vi "Target to Pixel.vi"(8 "Symbol":u32[][](array[colorbox]), 11 "Target Coordinates":dbl[](array[numeric])) -> (3 "Target Pixel":cluster{"X":i32, "Y":i32})   [LabVIEW 2018]
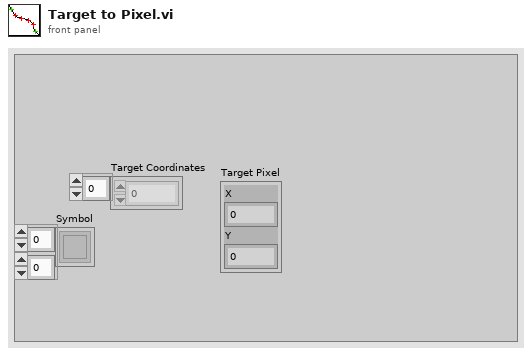
[diagram p1: front panel]
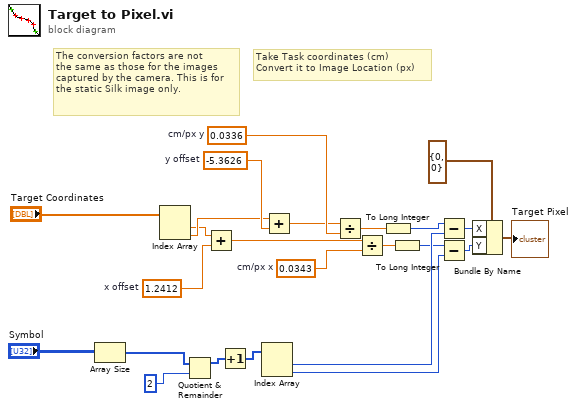
[diagram p0: block diagram]
diagram:
  w21 = 0.0336  # cm/px y
  w22 = 1.2412  # x offset
  w23 = 0.0343  # cm/px x
  w20 = -5.3626  # y offset
  # "The conversion factors are not \nthe same as those for the images\ncaptured by the camera. This is for\nthe static Silk image only."
  # "Take Task coordinates (cm)\nConvert it to Image Location (px)"
  n1 = Array Size(array="Symbol") -> (size(s)=w6:i32[])
  n2 = Index Array(array="Target Coordinates") -> (element #1=w1:dbl, element #2=w2:dbl)  [unwired: 2 in]
  n3 = Quotient & Remainder(x=w6, y=2) -> (x-y*floor(x/y)=w4:i32[])  [unwired: 1 out]
  n4 = Add(x=w1, y=w22) -> (x+y=w16:dbl)
  n5 = Increment(x=w4) -> (x+1=w3:i32[])
  n6 = Index Array(array=w3) -> (element #1=w10:i32, element #2=w7:i32)  [unwired: 2 in]
  n7 = Add(x=w2, y=w20) -> (x+y=w17:dbl)
  n8 = Divide(x=w17, y=w21) -> (x/y=w14:dbl)
  n9 = Divide(x=w16, y=w23) -> (x/y=w15:dbl)
  n10 = To Long Integer(number=w14) -> (32bit integer=w11:i32)
  n11 = To Long Integer(number=w15) -> (32bit integer=w9:i32)
  n12 = Subtract(x=w11, y=w10) -> (x-y=w12:i32)
  n13 = Subtract(x=w9, y=w7) -> (x-y=w8:i32)
  n14 = Bundle By Name(cluster=cluster{"X":i32, "Y":i32} {"X"=0, "Y"=0} ("Top Left Point"), "X"=w12, "Y"=w8) -> (→"Target Pixel":cluster{"X":i32, "Y":i32})
